vi "系统全局.vi"() -> ()   [LabVIEW 2016]
panel:
  in  "站点名称":string
  in  "CODmn":dbl
  in  "总氮":dbl
  in  "总磷":dbl
  in  "氨氮":dbl
  in  "浊度":dbl
  in  "比电导率":dbl
  in  "DOper":dbl
  in  "DO":dbl
  in  "pH":dbl
  in  "水温":dbl
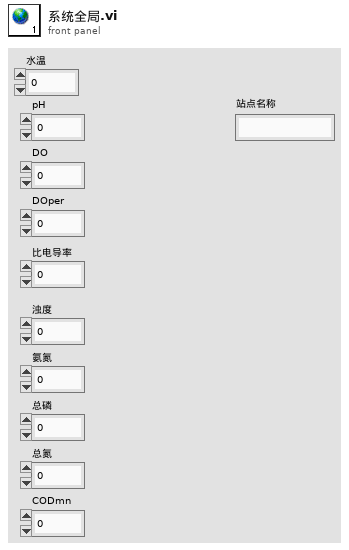
[diagram p1: front panel]
diagram:
